vi "setCmdDeterminer.vi"(8 "error in (no error)":errorcluster, 10 "Command Determiner":refnum<vi>, 11 "Subsystem in":refnum<class "Subsystem.lvclass">) -> (0 "error out":errorcluster, 2 "Updated?":bool, 3 "Subsystem out":refnum<class "Subsystem.lvclass">)   [LabVIEW 2017, in "Subsystem.lvclass"]
uses:
  <userlib>/836-Library/Robot/Subsystem/Subsystem.lvclass
  <userlib>/836-Library/Robot/Subsystem/Subsystem.lvclass/Subsystem.ctl
  <vilib>/Utility/error.llb/Error Cluster From Error Code.vi
  <vilib>/ErrorRing/Error Ring.xnode
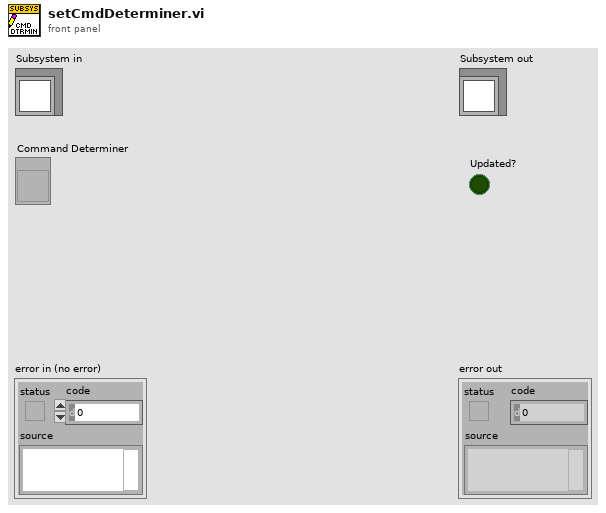
[diagram p1: front panel]
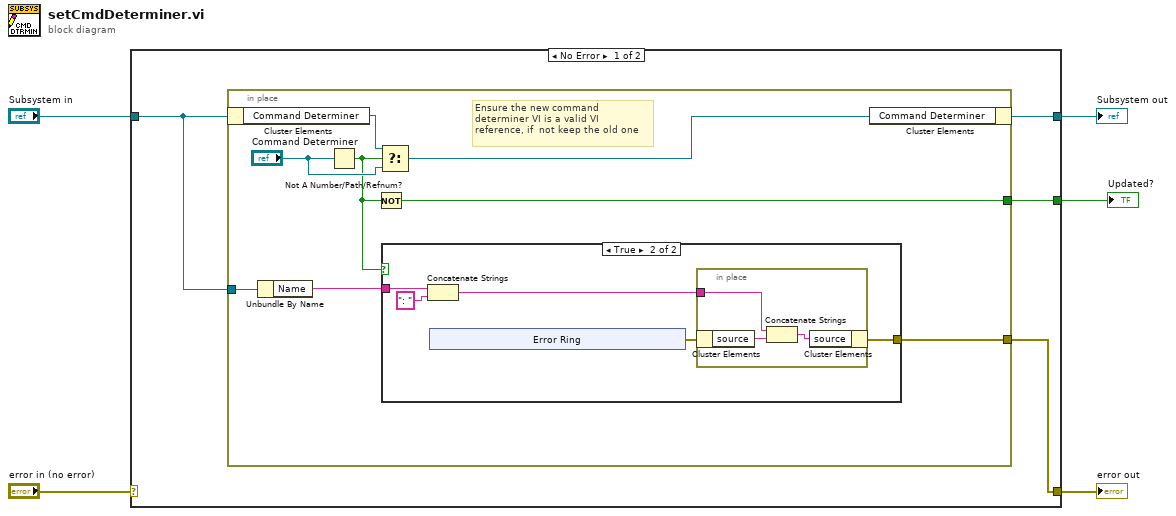
[diagram p0: block diagram]
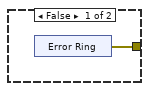
[diagram p2: hidden frame]
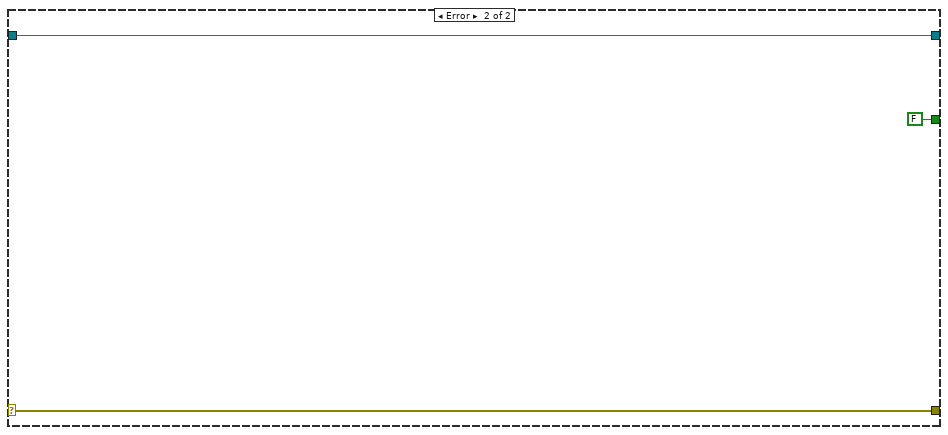
[diagram p3: hidden frame]
diagram:
  n1 = case shown="No Error" "error in (no error)" {
    selector: "error in (no error)" -> [_ w34]
    tunnel: [w6 w34] -> w4
    tunnel: [w9 w35] -> w2
    tunnel: "Subsystem in" -> [w8 w35]
    tunnel: [w7 FALSE] -> w1
    frame No Error {
      n2 = in-place {
        in-place-border: w8 -> [w14]
        in-place-border: [w13] -> w7
        in-place-border: [w11] -> w6
        # "Ensure the new command \ndeterminer VI is a valid VI \nreference, if  not keep the old one"
        n3 = in-place-cluster #1(w8) -> ("Command Determiner"=w17:refnum<vi>)
        n4 = Unbundle By Name(w14) -> ("Name"=w12:string)
        n5 = Not A Number/Path/Refnum?(number/path/refnum="Command Determiner") -> (NaN/Path/Refnum?=w10:bool)
        n6 = Not(x=w10) -> (.not. x?=w13:bool)
        n7 = Select(t=w17, s=w10, f="Command Determiner") -> (s? t:f=w15:refnum<vi>)
        n8 = case shown="True" w10 {
          tunnel: w12 -> [_ w23]
          tunnel: [w18 w20] -> w11
          frame False {
            n9 = xnode "Error Ring"() -> ("error out"=w18:errorcluster)
          }
          frame True {
            n10 = Concatenate Strings(w23, ": " ("string")) -> (w21:string)
            n11 = xnode "Error Ring"() -> ("error out"=w24:errorcluster)
            n12 = in-place {
              in-place-border: w21 -> [w25]
              n13 = in-place-cluster #2(w24) -> ("source"=w27:string)
              n14 = Concatenate Strings(w25, w27) -> (w26:string)
              n15 = in-place-cluster #2("source"=w26) -> (w20:errorcluster)
            }
          }
        }
        n16 = in-place-cluster #1("Command Determiner"=w15) -> (w9:refnum<class "Subsystem.lvclass">)
      }
    }
    frame Error {
    }
  }
  "error out" <- w4
  "Subsystem out" <- w2
  "Updated?" <- w1
